vi "first order system.vi"(8 "delta t":dbl=0.01 format="%.2f", 10 "a":dbl=1.0 format="%.2f", 11 "command":dbl=1.0 format="%.2f") -> (2 "response":dbl(graph)=-42.44427756719487)   [LabVIEW 2016]
doc: "This subVI mimics a first order system."
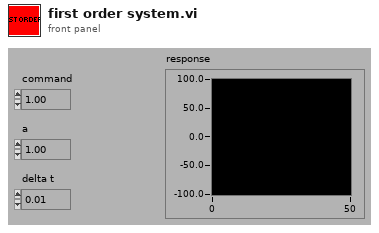
[diagram p1: front panel]
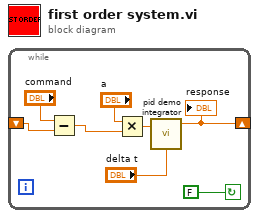
[diagram p0: block diagram]
diagram:
  n1 = while {
    shift-left: _ -> [w4]
    shift-right: [w7] -> _
    stop <- FALSE continue-if-true
    n2 = Subtract(x="command", y=w4) -> (x-y=w3:dbl)
    n3 = Multiply(x="a", y=w3) -> (x*y=w2:dbl)
    n4 = call "pid demo integrator.vi"("delta t"="delta t", "input"=w2) -> ("output"=w7:dbl)  [unwired: 3 in]
    "response" <- w7
  }
